vi "StartPCI.vi"(3 "error in (no error)":errorcluster, 6 "Device Number":i32) -> (0 "error out":errorcluster)   [LabVIEW 2015]
uses:
  BC637PCI.dll
panel:
  out "Result":i32
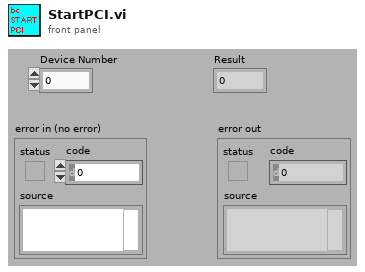
[diagram p1: front panel]
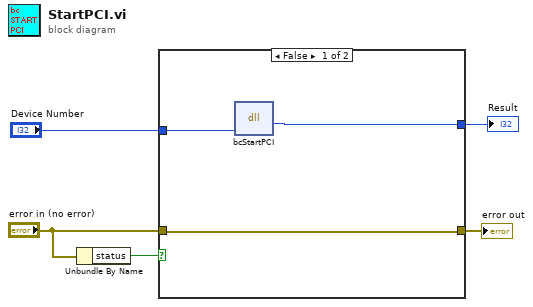
[diagram p0: block diagram]
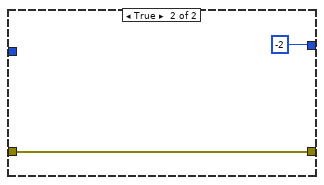
[diagram p2: hidden frame]
diagram:
  n1 = Unbundle By Name("error in (no error)") -> ("status"=w3:bool)
  n2 = case shown="False" w3 {
    tunnel: "Device Number" -> [w8 _]
    tunnel: "error in (no error)" -> [w6 w10]
    tunnel: [w6 w10] -> w2
    tunnel: [w7 -2] -> w1
    frame False {
      n3 = dll-call lib="C:/ALPHA GSCS/GSCS/Systems/SIcamera_Control/GPS_Drivers/BC637PCI.dll" fn="bcStartPCI"("devno"=w8) -> ("return type"=w7:i32)  [unwired: 4 in, 2 out]
    }
    frame True {
    }
  }
  "Result" <- w1
  "error out" <- w2
